vi "Actor Core.vi"(8 "error in":errorcluster, 11 "Example Source":refnum<class "Example Source.lvclass">) -> (0 "error out":errorcluster, 3 "Actor out":refnum<class "Actor.lvclass">)   [LabVIEW 2016, in "Example Source.lvlib" / "Example Source.lvclass"]
doc: "This is Actor Core.vi, the main message handling loop for Actors. An actor usually just sits in this loop and processes messages as they arrive. Any error returned by the message Do.vi call will stop the loop, with error code 43 as the cannonical signal to stop with no error sent to caller. Descendants may override that in Handle Error.vi."
uses:
  Example Source.lvclass
  C:/Projects/Shared Libraries/Event Actors/Event Source/Event Source.lvclass
  C:/Program Files (x86)/National Instruments/LabVIEW 2016/vi.lib/ActorFramework/Actor/Actor.lvclass
  <vilib>/ActorFramework/Actor/Actor.lvclass
  Event Source/Registerd Sinks.ctl
  Event Source/Sink Settings.ctl
  Example Source.lvclass/Example Source.ctl
  Event Source/Event Source.lvclass/Event Source.ctl
  <vilib>/ActorFramework/Actor/Actor.lvclass/Actor.ctl
  <vilib>/ActorFramework/Message Enqueuer/Message Enqueuer.lvclass/Message Enqueuer.ctl
  Example Events/Timestamp Event.lvclass
  C:/Projects/Shared Libraries/Event Actors/Event/Event.lvclass
  Event/Event.lvclass/Event.ctl
  Alternative Example Sink/Example Sink Messages/Update Time Msg/Update Time Msg.lvclass
  C:/Projects/Shared Libraries/Event Actors/Event Source Messages/Event Generated Msg/Event Generated Msg.lvclass
  Example Events/Double Array Event.lvclass
  Alternative Example Sink/Example Sink Messages/Update Array Msg/Update Array Msg.lvclass
  Write Boolean Notifier.vi
  Event Source/properties/Read Registered Sinks Event Ref.vi
  Event Source/properties/Read Sink Settings Event Ref.vi
  <vilib>/ActorFramework/Message Enqueuer/Init from Existing Queue.vi
  <vilib>/ActorFramework/Message Enqueuer/Enqueue.vi
  <vilib>/ActorFramework/Stop Msg/Stop Msg.lvclass
  C:/Program Files (x86)/National Instruments/LabVIEW 2016/vi.lib/ActorFramework/Message/Message.lvclass
  <vilib>/Utility/LVClass/Get LV Class Name.vi
  <resource>/AFDebug/Generate Trace for Message.vi
  <vilib>/ActorFramework/Message Priority Queue/Priority Enqueue.vi
  Timed Loop Controller/Timed Loop Controller/Timed Loop Controller.lvclass
  <vilib>/ActorFramework/Message Enqueuer/Message Enqueuer.lvclass
  Event/Event.lvclass
  Event Source Messages/Register by Name Msg/Register by Name Msg.lvclass
  Event Source Messages/Unregister by Name Msg/Unregister by Name Msg.lvclass
  Event Source Messages/Read Registered Sinks Msg/Read Registered Sinks Msg.lvclass
  Event Source/Event Source.lvclass
  Event Source Messages/Read Sink Settings Msg/Read Sink Settings Msg.lvclass
  Event Source Messages/Write Sink Settings Msg/Write Sink Settings Msg.lvclass
panel:
  in  "Sink Settings":T1
  in  "Write Sink Settings":bool
  in  "Read Sink Settings":bool
  out "Sink Settings Read":T1
  in  "Sink":T2
  out "Boolean Chart":i16(graph)
  in  "Registered for Data":bool=TRUE
  in  "Registered for Time":bool=TRUE
  in  "Stop Button":bool
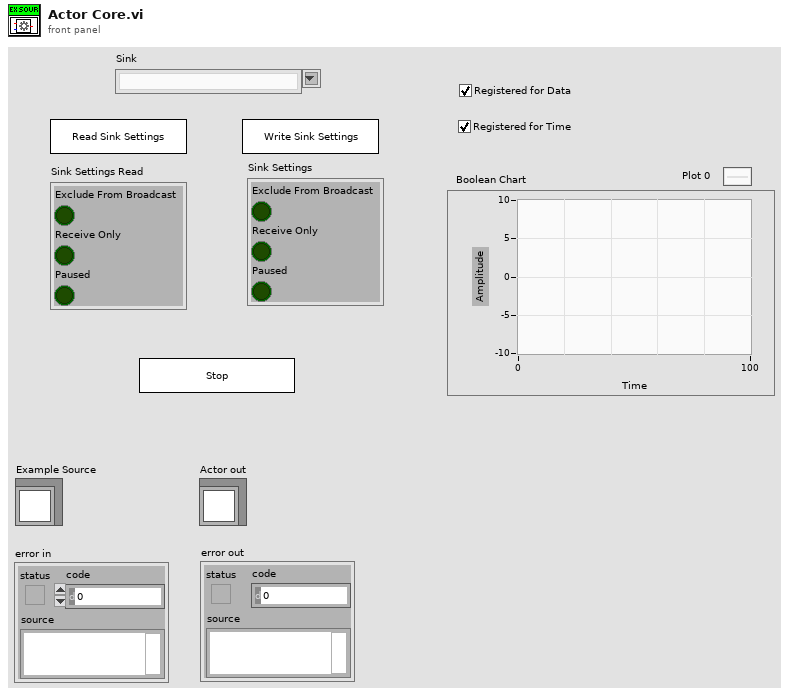
[diagram p1: front panel]
types:
  T1 = typedef "Event Source.lvlib/Event Source.lvclass/Sink Settings.ctl" = cluster{"Exclude From Broadcast":bool, "Receive Only":bool, "Paused":bool}
  T2 = typedef "Event Source.lvlib/Event Source.lvclass/Registerd Sinks.ctl" = string
  T3 = typedef "Event Source.lvlib/Event Source.lvclass/Registered Sinks Event Ref.ctl" = refnum<user-event>
  T4 = typedef "Event Source.lvlib/Event Source.lvclass/Sink Settings Event Ref.ctl" = refnum<user-event>
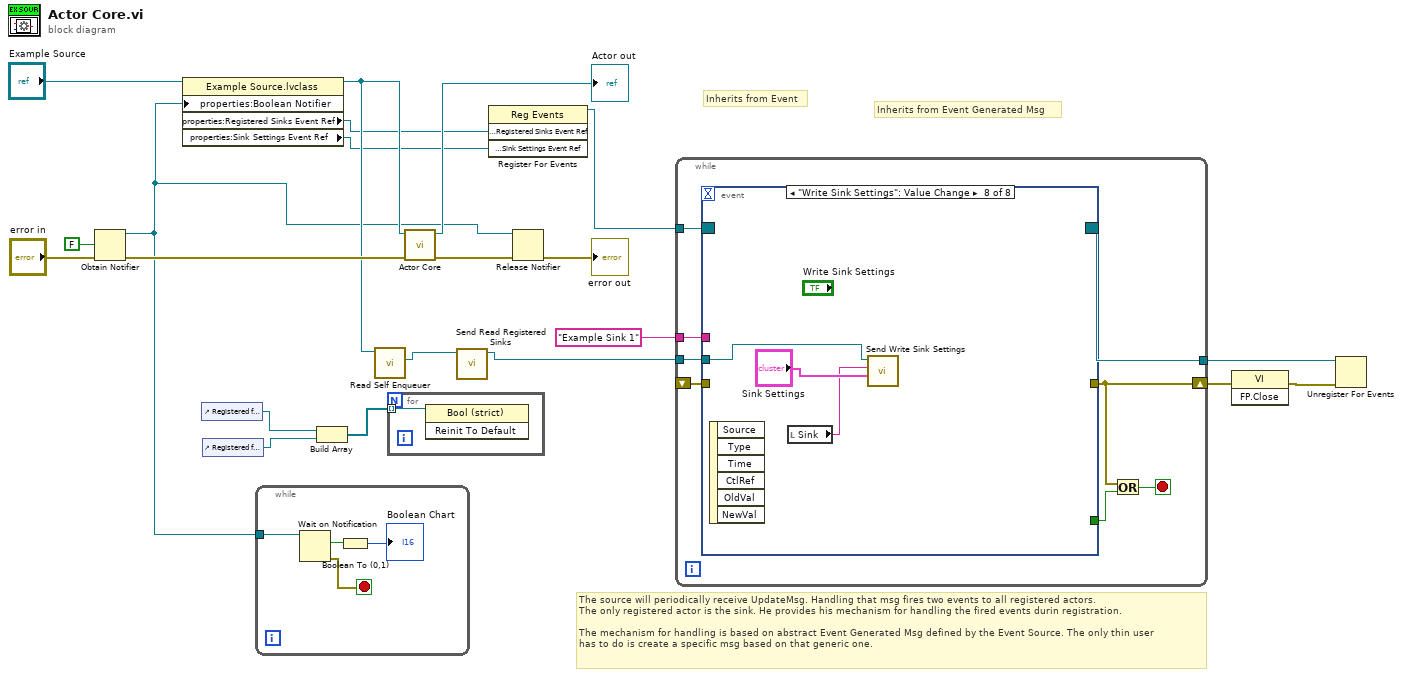
[diagram p0: block diagram]
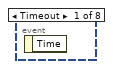
[diagram p2: hidden frame]
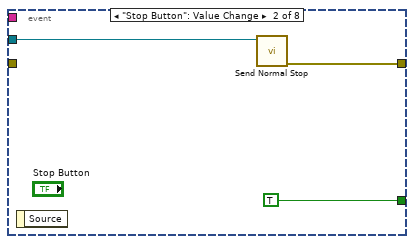
[diagram p3: hidden frame]
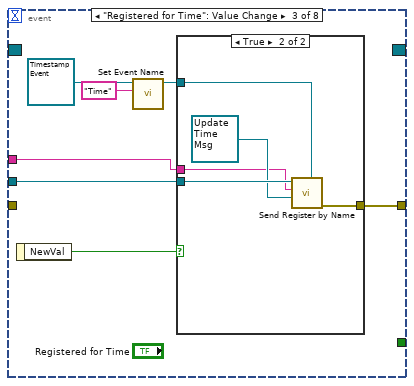
[diagram p4: hidden frame]
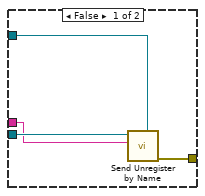
[diagram p5: hidden frame]
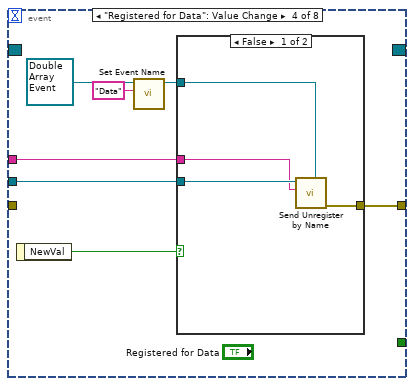
[diagram p6: hidden frame]
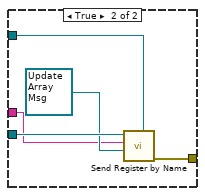
[diagram p7: hidden frame]
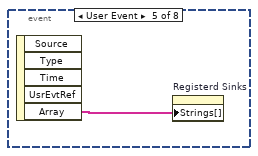
[diagram p8: hidden frame]
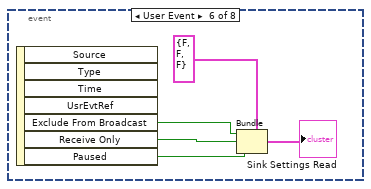
[diagram p9: hidden frame]
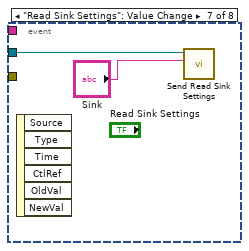
[diagram p10: hidden frame]
diagram:
  # "The source will periodically receive UpdateMsg. Handling that msg fires two events to all registered actors.\nThe only registered actor is the sink. He provides his mechanism for handling the fired events durin registration.\n\nThe mechanism for handling is based on abstract Event Generated Msg defined by the Event Source. The only thin user\nhas to do is create a specific msg based on that generic one."
  # "Inherits from Event"
  # "Inherits from Event Generated Msg"
  n1 = Obtain Notifier(notification data type=FALSE, error in (no error)="error in") -> (notifier out=w8:refnum<notifier>, error out=w11:errorcluster)  [unwired: 2 in, 1 out]
  n2 = property class="Example Source.lvclass"(reference="Example Source", "properties:Boolean Notifier"=w8) -> (reference out=w10:refnum<class "Example Source.lvclass">, "properties:Registered Sinks Event Ref"=w7:T3, "properties:Sink Settings Event Ref"=w6:T4)  [unwired: 1 in, 1 out]
  n3 = control-ref of="Registered for Time"() -> (w16:refnum<vi>)
  n4 = control-ref of="Registered for Data"() -> (w15:refnum<vi>)
  n5 = while {
    tunnel: w8 -> [w25]
    stop <- w22 stop-if-true
    n6 = Wait on Notification(notifier=w25) -> (notification=w24:bool, error out=w22:errorcluster)  [unwired: 3 in, 2 out]
    n7 = Boolean To (0,1)(Boolean=w24) -> (0, 1=→"Boolean Chart":i16)
  }
  n8 = Build Array(w16, w15) -> (w14:refnum<vi>[])
  n9 = call <vilib>:"Read Self Enqueuer.vi"("Actor"=w10) -> ("Self Enqueuer"=w4:refnum<class "Message Enqueuer.lvclass">)  [unwired: 10 in]
  n10 = for {
    tunnel: w14 -> [w26] mode=indexing
    n11 = invoke class="Bool (strict)" method="Reinit To Default"(reference=w26) -> ()  [unwired: 2 in, 3 out]
  }
  n12 = call-parent "Actor Core.vi"("error in"=w11, "Timed Loop Controller"=w10) -> ("error out"=w21:errorcluster, "Actor out"=→"Actor out":refnum<class "Actor.lvclass">)  [unwired: 8 in]
  n13 = call "Send Read Registered Sinks.vi"("Message Enqueuer in"=w4) -> ("Message Enqueuer out"=w3:refnum<class "Message Enqueuer.lvclass">)  [unwired: 9 in, 1 out]
  n14 = register-events(w7, w6) -> (reference out=w5:refnum<event-registration>)  [unwired: 2 in, 1 out]
  n15 = Release Notifier(notifier=w8, error in (no error)=w21) -> (error out=→"error out":errorcluster)  [unwired: 1 in, 2 out]
  n16 = while {
    tunnel: w3 -> [w33]
    shift-right: [w31] -> w19
    shift-left: _ -> [w34]
    tunnel: "Example Sink 1" ("Debug Alias") -> [w29]
    tunnel: w5 -> [w28]
    tunnel: [w27] -> w1
    stop <- w30 stop-if-true
    n17 = event shown="[7] \"Write Sink Settings\": Value Change" {
      selector: w28 -> [_ _ _ _ _ _ _ _]
      dyn-events: [_ _ _ _ _ _ _ _] -> w27
      timeout: _ -> [_ _ _ _ _ _ _ _]
      tunnel: w34 -> [_ _ _ _ _ _ _ _]
      tunnel: w33 -> [_ w36 w43 w59 _ _ w77 w78]
      tunnel: [_ w37 w42 w58 _ _ _ _] -> w31
      tunnel: [_ TRUE _ _ _ _ _ _] -> w32
      tunnel: w29 -> [_ _ w38 w54 _ _ _ _]
      event Timeout {
        n18 = event-data() -> ()  [unwired: 1 in, 1 out]
      }
      event "Stop Button": Value Change {
        n19 = event-data() -> ()  [unwired: 1 in, 1 out]
        n20 = call <vilib>:"Send Normal Stop.vi"("Message Enqueuer"=w36) -> ("error out"=w37:errorcluster)  [unwired: 10 in]
      }
      event "Registered for Time": Value Change {
        n21 = event-data() -> ("NewVal"=w44:bool)  [unwired: 1 in]
        n22 = call "Set Event Name.vi"("Name (Generic)"="Time", "Event In"=refnum<class "Timestamp Event.lvclass"> refnum ("Timestamp Event.lvclass")) -> ("Event Out"=w39:refnum<class "Timestamp Event.lvclass">)  [unwired: 9 in]
        n23 = case shown="True" w44 {
          tunnel: w43 -> [w48 w53]
          tunnel: w39 -> [w47 w51]
          tunnel: [w46 w50] -> w42
          tunnel: w38 -> [w45 w49]
          frame False {
            n24 = call "Send Unregister by Name.vi"("Event"=w47, "Sink Name"=w45, "Message Enqueuer in"=w48) -> ("error out"=w46:errorcluster)  [unwired: 7 in, 1 out]
          }
          frame True {
            n25 = call "Send Register by Name.vi"("Event"=w51, "Event Fire Handler"=refnum<class "Update Time Msg.lvclass"> refnum ("Update Time Msg.lvclass"), "Sink Name"=w49, "Message Enqueuer in"=w53) -> ("error out"=w50:errorcluster)  [unwired: 6 in, 1 out]
          }
        }
      }
      event "Registered for Data": Value Change {
        n26 = event-data() -> ("NewVal"=w60:bool)  [unwired: 1 in]
        n27 = call "Set Event Name.vi"("Name (Generic)"="Data", "Event In"=refnum<class "Double Array Event.lvclass"> refnum ("Double Array Event.lvclass")) -> ("Event Out"=w56:refnum<class "Double Array Event.lvclass">)  [unwired: 9 in]
        n28 = case shown="False" w60 {
          tunnel: w59 -> [w64 w69]
          tunnel: w56 -> [w63 w68]
          tunnel: [w62 w67] -> w58
          tunnel: w54 -> [w61 w65]
          frame False {
            n29 = call "Send Unregister by Name.vi"("Event"=w63, "Sink Name"=w61, "Message Enqueuer in"=w64) -> ("error out"=w62:errorcluster)  [unwired: 7 in, 1 out]
          }
          frame True {
            n30 = call "Send Register by Name.vi"("Event"=w68, "Event Fire Handler"=refnum<class "Update Array Msg.lvclass"> refnum ("Update Array Msg.lvclass"), "Sink Name"=w65, "Message Enqueuer in"=w69) -> ("error out"=w67:errorcluster)  [unwired: 6 in, 1 out]
          }
        }
      }
      event User Event {
        n31 = event-data() -> ("Array"=w70:string[])  [unwired: 1 in, 4 out]
        n32 = property on="Registerd Sinks" class="CmbBox (strict)"("Strings[]"=w70) -> ()  [unwired: 2 in, 2 out]
      }
      event User Event {
        n33 = event-data() -> ("Exclude From Broadcast"=w74:bool, "Receive Only"=w73:bool, "Paused"=w72:bool)  [unwired: 1 in, 4 out]
        n34 = Bundle(cluster=T1 {"Exclude From Broadcast"=FALSE, "Receive Only"=FALSE, "Paused"=FALSE} ("Sink Settings"), "Exclude From Broadcast"=w74, "Receive Only"=w73, "Paused"=w72) -> (→"Sink Settings Read":T1)
      }
      event "Read Sink Settings": Value Change {
        n35 = event-data() -> ()  [unwired: 1 in, 6 out]
        n36 = call "Send Read Sink Settings.vi"("Sink Name"="Sink", "Message Enqueuer in"=w77) -> ()  [unwired: 8 in, 2 out]
      }
      event "Write Sink Settings": Value Change {
        n37 = event-data() -> ()  [unwired: 1 in, 6 out]
        n38 = local read "Sink"() -> (w79:T2)
        n39 = call "Send Write Sink Settings.vi"("Sink Settings"="Sink Settings", "Sink Name"=w79, "Message Enqueuer in"=w78) -> ()  [unwired: 7 in, 2 out]
      }
    }
    n40 = Or(x=w31, y=w32) -> (x .or. y?=w30:bool)
  }
  n41 = invoke class="VI" method="FP.Close"(error in=w19) -> (error out=w2:errorcluster)  [unwired: 2 in, 2 out]
  n42 = Unregister For Events(event registration refnum=w1, error in=w2) -> ()  [unwired: 1 out]
